vi "setState.vi"(8 "error in (no error)":errorcluster, 10 "Output":T1, 11 "Inst.RP100 in":refnum<class "Inst.RP100.lvclass">) -> (0 "error out":errorcluster, 3 "Inst.RP100 out":refnum<class "Inst.RP100.lvclass">)   [LabVIEW 2019, in "Inst.RP100.lvlib" / "Inst.RP100.lvclass"]
doc: "Set the output <b>Level</b> with <b>Slew</b> rate on the selected <b>Output Channel</b>"
uses:
  Inst.RP100.lvclass
  Typedefs/State--Enum.ctl
  Typedefs/Inst.RP100.Commands--Enum.ctl
  Typedefs/setState--Cluster.ctl
  bd6c3626-3ffe-41a5-babe-17ac00828b50.vi
  bd6c3626-3ffe-41a5-babe-17ac00828b50.vi/b3718d6e-7fad-4f42-a04f-1bb3c5c40f3e.vi
  bd6c3626-3ffe-41a5-babe-17ac00828b50.vi/b3718d6e-7fad-4f42-a04f-1bb3c5c40f3e.vi/9bd04e1a-d99a-45f8-9a48-64089f0a925a.vi
  bd6c3626-3ffe-41a5-babe-17ac00828b50.vi/b3718d6e-7fad-4f42-a04f-1bb3c5c40f3e.vi/5be528f3-3fe2-49cf-9e7b-580a7b495766.vi
  <vilib>/Utility/Data Type/Get Type Information.vi
  <vilib>/JDP Science/JSONtext/JSON text to Variant.vi
  <vilib>/JDP Science/JSONtext/LVClass Serializer/JSONtext LVClass Serializer.lvclass
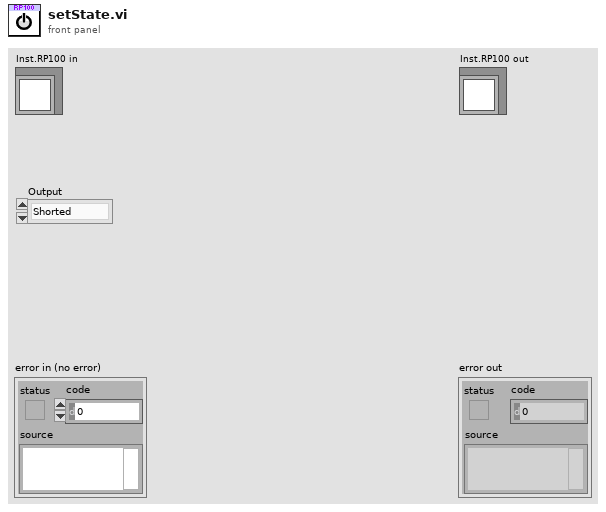
[diagram p1: front panel]
types:
  T1 = typedef "Inst.RP100.lvlib/Inst.RP100.lvclass/State--Enum.ctl" = enum16{"Shorted", "Enabled"}
  T2 = typedef "Inst.RP100.lvlib/Inst.RP100.lvclass/setState--Cluster.ctl" = cluster{"State":T1}
  T3 = typedef "Inst.RP100.lvlib/Inst.RP100.lvclass/Inst.RP100.Commands--Enum.ctl" = enum16{"setState", "setLevel", "getLevel"}
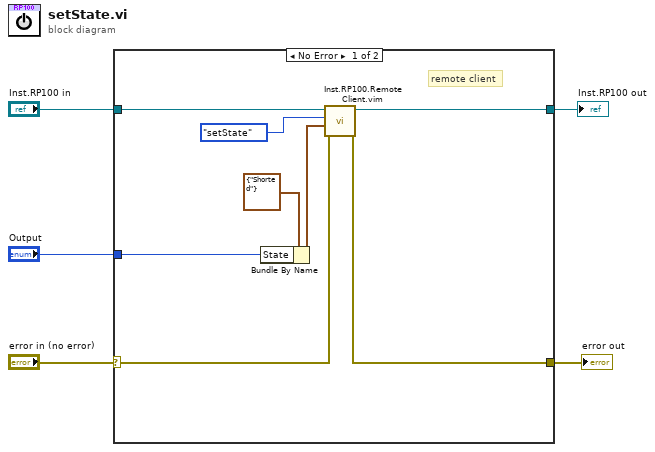
[diagram p0: block diagram]
diagram:
  n1 = case shown="No Error" "error in (no error)" {
    selector: "error in (no error)" -> [w12 w15]
    tunnel: [w11 w15] -> w4
    tunnel: "Output" -> [w10 _]
    tunnel: "Inst.RP100 in" -> [w8 w14]
    tunnel: [w13 w14] -> w1
    frame No Error {
      # "remote client"
      n2 = Bundle By Name(cluster=T2 {"State"=enum."Shorted"} ("setOutput"), "State"=w10) -> (w6:T2)
      n3 = call "Inst.RP100.Remote Client.vim"("error in (no error)"=w12, "params"=w6, "Commands"=Inst.RP100.Commands--Enum."setState", "Inst.RP100 in"=w8) -> ("error out"=w11:errorcluster, "Inst.RP100 out"=w13:refnum<class "Inst.RP100.lvclass">)  [unwired: 5 in, 1 out]
    }
    frame Error {
    }
  }
  "error out" <- w4
  "Inst.RP100 out" <- w1
